vi "Msg Send Priority Message.vi"   [LabVIEW 2014]
doc: "Sends a high priority message to the front specified message queue (or event structure). This function awaits a response from the recipient which should be sent with Msg Send Response.vi.\n\nThis is part of the Msg suite, intended to make messaging architectures in LabVIEW\nSee the template \"Message Based Application Template.vi\" for normal usage.\n\nCopyright 2005-2016 Jason Sommerville\n\nSends a response to the original sender of a message (sent via Msg Send Message). It should form bookends with Msg Get Message in the message handling loop.\n\nThis is part of the Msg suite, intended to make messaging architectures in LabVIEW\nSee the template \"Message Based Application Template.vi\" for normal usage.\n\nCopyright 2005-2016 Jason Sommerville\n\nThis VI may be freely used, modified or distributed under the BSD license."
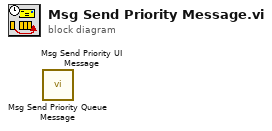
[diagram p0: block diagram]
diagram:
  n1 = call "Msg Send Priority Queue Message.vi"() -> ()  [unwired: 7 in, 3 out]
  n2 = call "Msg Send Priority UI Message.vi"() -> ()  [unwired: 8 in, 2 out]
